vi "Mux.vi"(0 "write command":T3, 1 "retrieve data fifo size":u8, 5 "read command":T2, 7 "completed read request":bool, 12 "ready for output":bool) -> (4 "command":T1, 6 "write is pending (1 cycle early)":bool, 8 "retrieve fifo full (1 cycle early)":bool)   [LabVIEW 2011, in "niRFRIO SRAM 1.0.0 FPGA.lvlib"]
uses:
  <instrlib>/RF-RIO/SRAM/1.0.0/FPGA/niRFRIO SRAM 1.0.0 FPGA.lvlib
  <instrlib>/RF-RIO/SRAM/1.0.0/FPGA/Private/Write Command.ctl
  <instrlib>/RF-RIO/SRAM/1.0.0/FPGA/Private/Read Command.ctl
  <instrlib>/RF-RIO/SRAM/1.0.0/FPGA/Private/Command.ctl
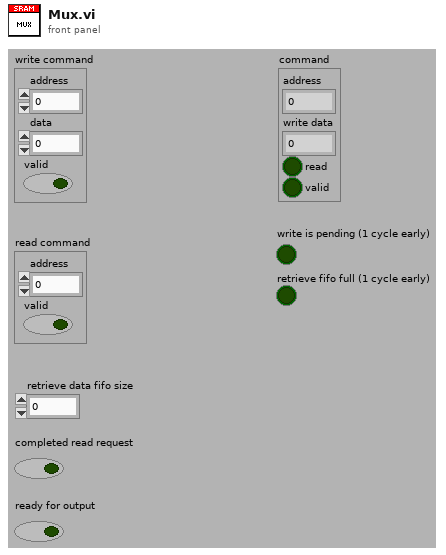
[diagram p1: front panel]
types:
  T1 = typedef "niRFRIO SRAM 1.0.0 FPGA.lvlib/Command.ctl" = cluster{"address":u32, "write data":u64, "read":bool, "valid":bool}
  T2 = typedef "niRFRIO SRAM 1.0.0 FPGA.lvlib/Read Command.ctl" = cluster{"address":u32, "valid":bool}
  T3 = typedef "niRFRIO SRAM 1.0.0 FPGA.lvlib/Write Command.ctl" = cluster{"address":u32, "data":u64, "valid":bool}
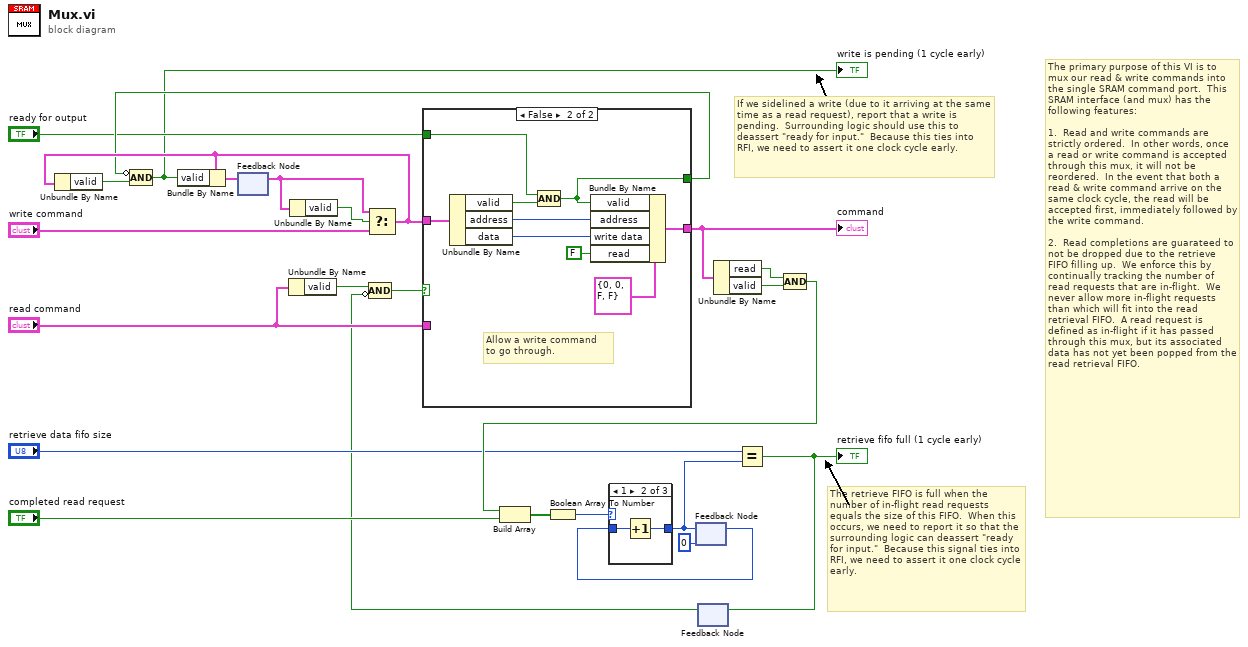
[diagram p0: block diagram]
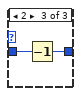
[diagram p3: hidden frame]
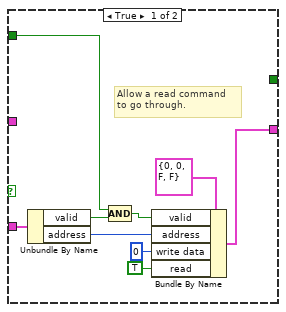
[diagram p4: hidden frame]
diagram:
  # "The retrieve FIFO is full when the number of in-flight read requests equals the size of this FIFO.  When this occurs, we need to report it so that the surrounding logic can deassert \"ready for input.\"  Because this signal ties into RFI, we need to assert it one clock cycle early."
  # "If we sidelined a write (due to it arriving at the same time as a read request), report that a write is pending.  Surrounding logic should use this to deassert \"ready for input.\"  Because this ties into RFI, we need to assert it one clock cycle early."
  # "The primary purpose of this VI is to mux our read & write commands into the single SRAM command port.  This SRAM interface (and mux) has the following features:\n\n1.  Read and write commands are strictly ordered.  In other words, once a read or write command is accepted through this mux, it will not be reordered.  In the event that both a read & write command arrive on the same clock cycle, the read will be accepted first, immediately followed by the write command.\n\n2.  Read completions are guarateed to not be dropped due to the retrieve FIFO filling up.  We enforce this by continually tracking the number of read requests that are in-flight.  We never allow more in-flight requests than which will fit into the read retrieval FIFO.  A read request is defined as in-flight if it has passed through this mux, but its associated data has not yet been popped from the read retrieval FIFO."
  n1 = feedback #1() -> (w22:T3)  [unwired: 1 in]
  n2 = Unbundle By Name("read command") -> ("valid"=w17:bool)
  n3 = Unbundle By Name(w22) -> ("valid"=w1:bool)
  n4 = Select(t=w22, s=w1, f="write command") -> (s? t:f=w21:T3)
  n5 = Unbundle By Name(w21) -> ("valid"=w23:bool)
  n6 = feedback #2(u8 0) -> (w6:u8)
  n7 = feedback #3() -> (w2:bool)  [unwired: 1 in]
  n8 = Compound Arithmetic op=AND(w17, invert w2) -> (w16:bool)
  n9 = case shown="False" w16 {
    tunnel: w21 -> [_ w43]
    tunnel: "read command" -> [w32 _]
    tunnel: [w33 w38] -> w13
    tunnel: [_ w36] -> w20
    tunnel: "ready for output" -> [w26 w35]
    frame True {
      # "Allow a read command\nto go through."
      n10 = Unbundle By Name(w32) -> ("valid"=w28:bool, "address"=w31:u32)
      n11 = Compound Arithmetic op=AND(w26, w28) -> (w27:bool)
      n12 = Bundle By Name(cluster=T1 {"address"=0, "write data"=0, "read"=FALSE, "valid"=FALSE} ("command"), "valid"=w27, "address"=w31, "write data"=u64 0, "read"=TRUE ("valid")) -> (w33:T1)
    }
    frame False {
      # "Allow a write command\nto go through."
      n13 = Unbundle By Name(w43) -> ("valid"=w37:bool, "address"=w41:u32, "data"=w40:u64)
      n14 = Compound Arithmetic op=AND(w35, w37) -> (w36:bool)
      n15 = Bundle By Name(cluster=T1 {"address"=0, "write data"=0, "read"=FALSE, "valid"=FALSE} ("command"), "valid"=w36, "address"=w41, "write data"=w40, "read"=FALSE ("write")) -> (w38:T1)
    }
  }
  "command" <- w13
  n16 = Compound Arithmetic op=AND(invert w20, w23) -> (w15:bool)
  "write is pending (1 cycle early)" <- w15
  n17 = Bundle By Name(cluster=w21, "valid"=w15) -> (w24:T3)
  n18 = feedback-in #1(w24) -> ()
  n19 = Unbundle By Name(w13) -> ("read"=w12:bool, "valid"=w11:bool)
  n20 = Compound Arithmetic op=AND(w12, w11) -> (w10:bool)
  n21 = Build Array(w10, "completed read request") -> (w8:bool[])
  n22 = Boolean Array To Number(Boolean array=w8) -> (number=w7:u8)
  n23 = case shown="1" w7 {
    tunnel: w6 -> [w44 w46 w48]
    tunnel: [w44 w45 w47] -> w4
    frame 0, 3, Default {
    }
    frame 1 {
      n24 = Increment(x=w46) -> (x+1=w45:u8)
    }
    frame 2 {
      n25 = Decrement(x=w48) -> (x-1=w47:u8)
    }
  }
  n26 = feedback-in #2(w4) -> ()
  n27 = Equal?(x="retrieve data fifo size", y=w4) -> (x = y?=w3:bool)
  "retrieve fifo full (1 cycle early)" <- w3
  n28 = feedback-in #3(w3) -> ()
